vi "Varient_Current_Status.vi"(5 "Currenrt Varient path":path, 7 "Enum":enum16{"Write", "Read"}(ring), 8 "error in":errorcluster, 9 "AUTO/MANUAL":string="CURRENT_VARIENT", 10 "Batch Size":i32, 11 "Varient count":i32) -> (0 "error out":errorcluster, 1 "Batch Size":i32, 2 "Varient Count":i32)   [LabVIEW 2017]
uses:
  <vilib>/Utility/config.llb/Write Key (I32).vi
  <vilib>/Utility/config.llb/Read Key (I32).vi
  <vilib>/Utility/config.llb/NI_LVConfig.lvlib
panel:
  # "Varient Current Status & Count"
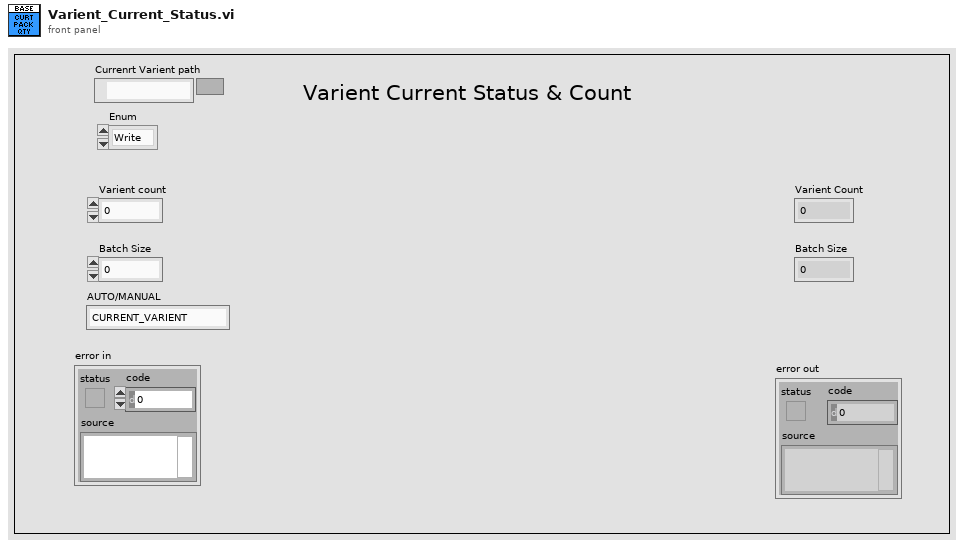
[diagram p1: front panel]
types:
  T1 = typedef "NI_LVConfig.lvlib/Config Data RefNum.ctl" = refnum<k1>
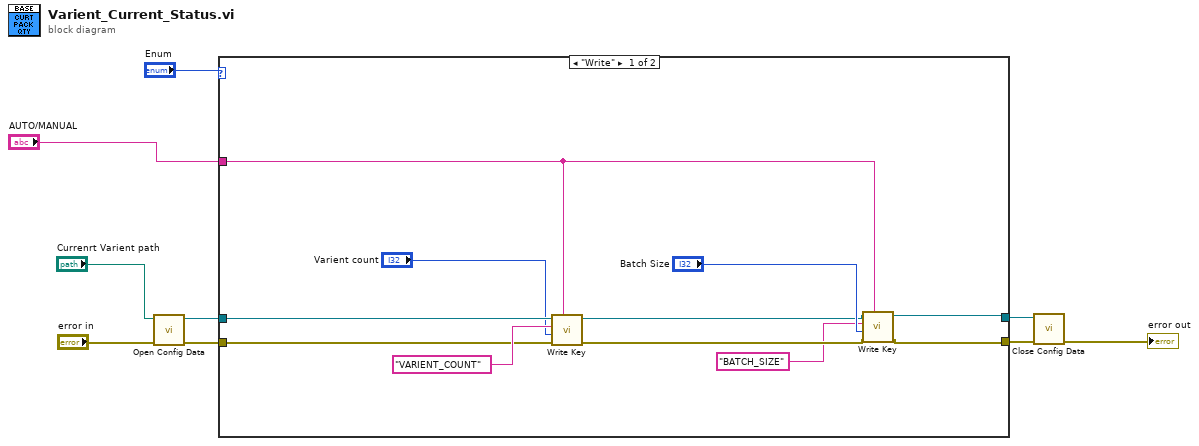
[diagram p0: block diagram]
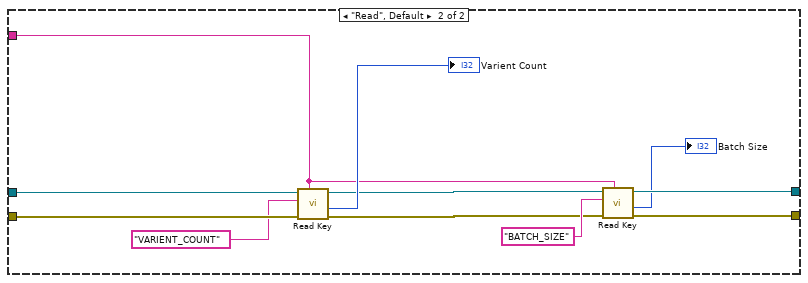
[diagram p2: hidden frame]
diagram:
  n1 = call <vilib>:"Open Config Data.vi"("error in (no error)"="error in", "configuration file path"="Currenrt Varient path") -> ("error out"=w8:errorcluster, "refnum"=w9:T1)  [unwired: 7 in, 1 out]
  n2 = case shown="\"Write\"" "Enum" {
    tunnel: w9 -> [w18 w31]
    tunnel: w8 -> [w19 w30]
    tunnel: [w14 w26] -> w5
    tunnel: [w12 w24] -> w4
    tunnel: "AUTO/MANUAL" -> [w10 w21]
    frame "Write" {
      n3 = call-poly <vilib>:"Write Key.vi"("section"=w10, "error in (no error)"=w19, "value"="Varient count", "key"="VARIENT_COUNT" ("name or relative path"), "refnum"=w18) -> ("error out"=w15:errorcluster, "refnum out"=w13:T1)  [unwired: 4 in, 1 out]
      n4 = call-poly <vilib>:"Write Key.vi"("section"=w10, "error in (no error)"=w15, "value"="Batch Size", "key"="BATCH_SIZE" ("name or relative path"), "refnum"=w13) -> ("error out"=w14:errorcluster, "refnum out"=w12:T1)  [unwired: 4 in, 1 out]
    }
    frame "Read", Default {
      n5 = call-poly <vilib>:"Read Key.vi"("section"=w21, "error in (no error)"=w30, "key"="VARIENT_COUNT" ("name or relative path"), "refnum"=w31) -> ("error out"=w27:errorcluster, "value"=→"Varient Count":i32, "refnum out"=w25:T1)  [unwired: 4 in, 1 out]
      n6 = call-poly <vilib>:"Read Key.vi"("section"=w21, "error in (no error)"=w27, "key"="BATCH_SIZE" ("name or relative path"), "refnum"=w25) -> ("error out"=w26:errorcluster, "value"=→"Batch Size":i32, "refnum out"=w24:T1)  [unwired: 4 in, 1 out]
    }
  }
  n7 = call <vilib>:"Close Config Data.vi"("error in (no error)"=w5, "refnum"=w4) -> ("error out"=→"error out":errorcluster)  [unwired: 8 in, 1 out]
